vi "getAllSpectraFromFolder.vi"(11 "Spectra Folder::":path) -> (2 "spectra":dbl[][][](array[numeric]) caption="spectrum\n\n\nFrequency\n\n\nColumn")   [LabVIEW 2021]
uses:
  92a57d49-5429-4118-b928-33e5c23aece6.vi
  <vilib>/Comparison/Less/Less Functor/Less Functor.lvclass
panel:
  in  "OK Button":bool
  in  "chooseSpectra:":i32[](listbox)
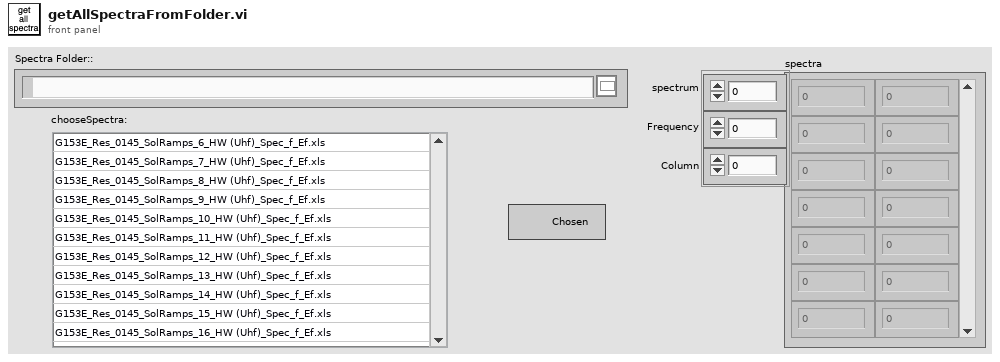
[diagram p1: front panel]
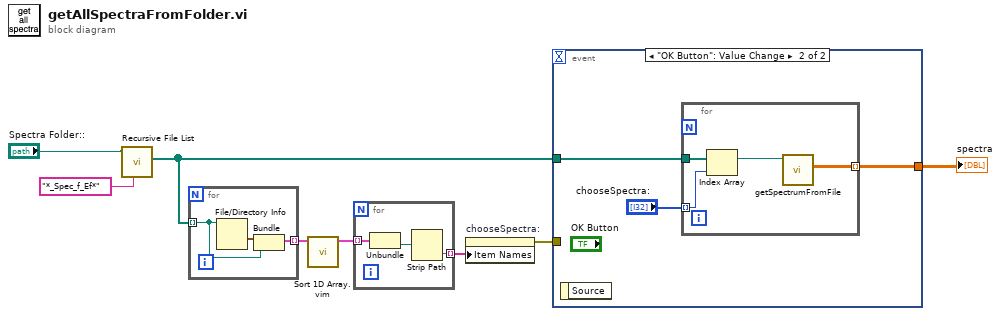
[diagram p0: block diagram]
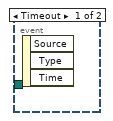
[diagram p2: hidden frame]
diagram:
  n1 = call <vilib>:"Recursive File List.vi"("pattern"="*_Spec_f_Ef*", "Folder Path"="Spectra Folder::") -> ("All Files in Dir"=w3:path[])  [unwired: 5 in, 4 out]
  n2 = for {
    tunnel: w3 -> [w10] mode=indexing
    tunnel: [w9] -> w1 mode=indexing
    n3 = File/Directory Info(path=w10) -> (last mod=w11:timestamp)  [unwired: 1 in, 6 out]
    n4 = Bundle("last mod"=w11, w10) -> (w9:cluster{"last mod":timestamp, path})  [unwired: 1 in]
  }
  n5 = call "Sort 1D Array.vim"("unsorted array"=w1) -> ("sorted array"=w2:cluster{"last mod":timestamp, path}[])  [unwired: 10 in]
  n6 = for {
    tunnel: w2 -> [w14] mode=indexing
    tunnel: [w13] -> w5 mode=indexing
    n7 = Unbundle(w14) -> (w12:path)  [unwired: 1 out]
    n8 = Strip Path(path=w12) -> (name=w13:string)  [unwired: 1 out]
  }
  n9 = property on="chooseSpectra:" class="LstBox (strict)"("Item Names"=w5) -> (error out=w4:errorcluster)  [unwired: 2 in, 1 out]
  n10 = event shown="[1] \"OK Button\": Value Change" {
    selector: _ -> [_ _]
    dyn-events: _ -> [_ _]
    timeout: _ -> [_ _]
    tunnel: [_ w15] -> w7
    tunnel: w3 -> [_ w16]
    tunnel: w4 -> [_ _]
    event Timeout {
      n11 = event-data() -> ()  [unwired: 1 in, 3 out]
    }
    event "OK Button": Value Change {
      n12 = event-data() -> ()  [unwired: 1 in, 1 out]
      n13 = for {
        tunnel: w16 -> [w20]
        tunnel: [w21] -> w15 mode=indexing
        tunnel: "chooseSpectra:" -> [w18] mode=indexing
        n14 = Index Array(array=w20, index=w18) -> (element=w19:path)
        n15 = call "getSpectrumFromFile.vi"("File Path Control"=w19) -> ("array"=w21:dbl[][])  [unwired: 10 in]
      }
    }
  }
  "spectra" <- w7
